vi "programa14.vi"() -> ()   [LabVIEW 2011]
panel:
  in  "stop":bool
  out "Velocidad":i32(knob) scale=0.0..180.0
  in  "Reducir":bool
  in  "Aumentar":bool
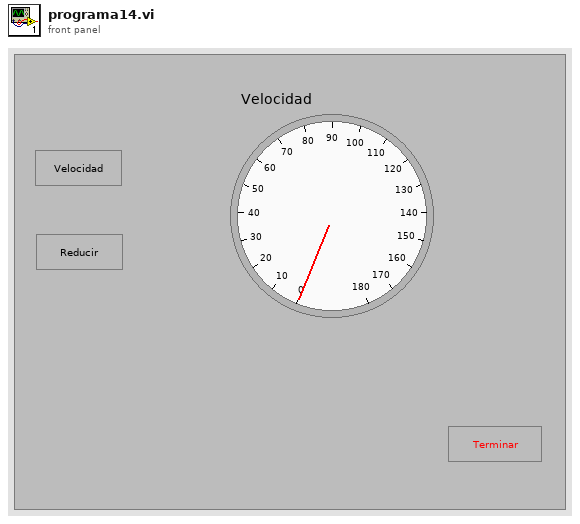
[diagram p1: front panel]
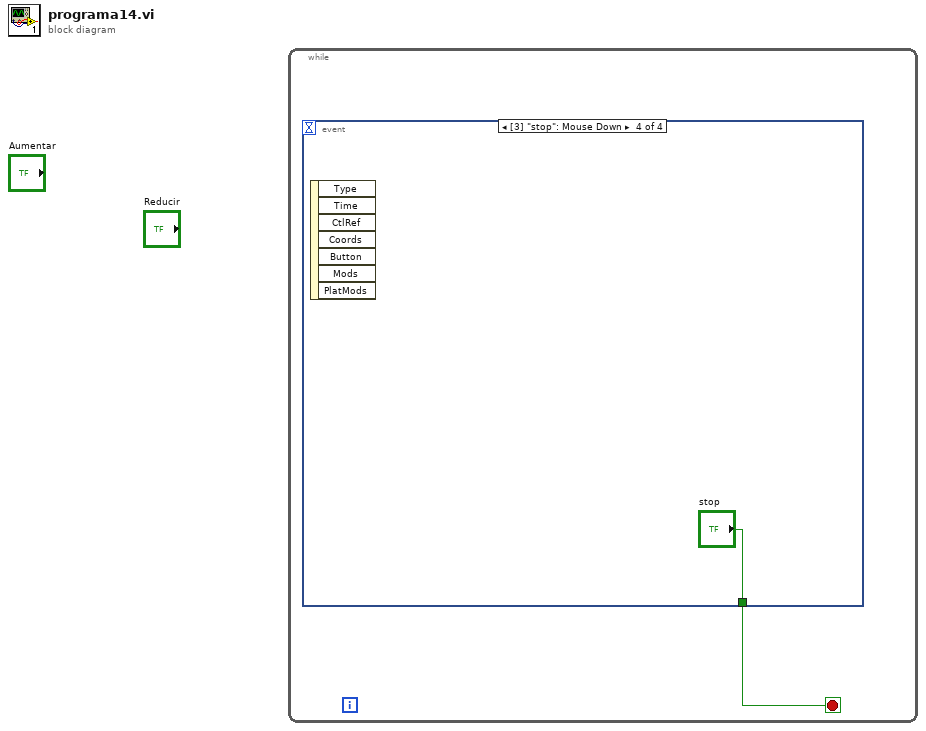
[diagram p0: block diagram]
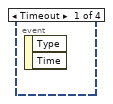
[diagram p2: hidden frame]
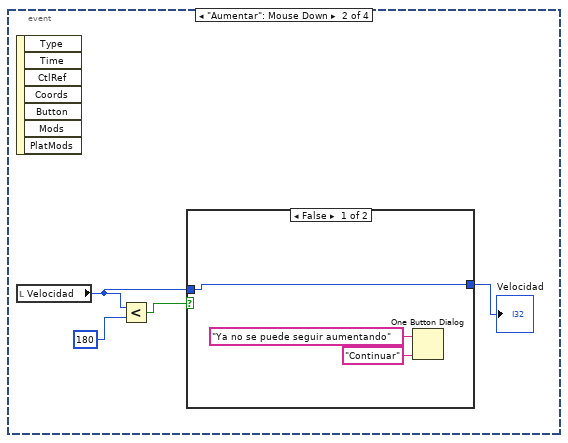
[diagram p3: hidden frame]
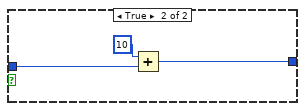
[diagram p4: hidden frame]
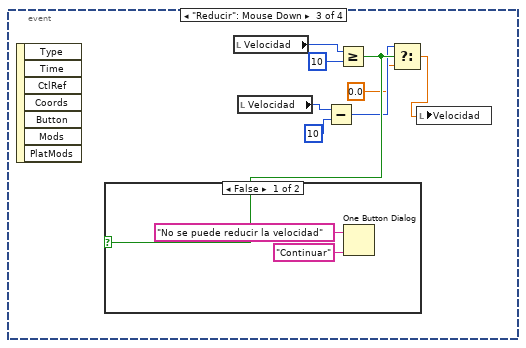
[diagram p5: hidden frame]
diagram:
  n1 = while {
    stop <- w1 stop-if-true
    n2 = event shown="[3] \"stop\": Mouse Down" {
      selector: _ -> [_ _ _ _]
      dyn-events: _ -> [_ _ _ _]
      timeout: _ -> [_ _ _ _]
      tunnel: [_ _ _ "stop"] -> w1
      event Timeout {
        n3 = event-data() -> ()  [unwired: 1 in, 2 out]
      }
      event "Aumentar": Mouse Down {
        n4 = event-data() -> ()  [unwired: 1 in, 7 out]
        n5 = local read "Velocidad"() -> (w4:i32)
        n6 = Less?(x=w4, y=180) -> (x < y?=w3:bool)
        n7 = case shown="False" w3 {
          tunnel: [w8 w10] -> w5
          tunnel: w4 -> [w8 w9]
          frame False {
            n8 = One Button Dialog(message="Ya no se puede seguir aumentando", button name ("OK")="Continuar") -> ()  [unwired: 1 out]
          }
          frame True {
            n9 = Add(x=10, y=w9) -> (x+y=w10:i32)
          }
        }
        "Velocidad" <- w5
      }
      event "Reducir": Mouse Down {
        n10 = event-data() -> ()  [unwired: 1 in, 7 out]
        n11 = local read "Velocidad"() -> (w15:i32)
        n12 = local read "Velocidad"() -> (w18:i32)
        n13 = Subtract(x=w18, y=10) -> (x-y=w13:i32)
        n14 = Greater Or Equal?(x=w15, y=10) -> (x >= y?=w14:bool)
        n15 = case shown="False" w14 {
          frame False {
            n16 = One Button Dialog(message="No se puede reducir la velocidad", button name ("OK")="Continuar") -> ()  [unwired: 1 out]
          }
          frame True {
          }
        }
        n17 = Select(t=w13, s=w14, f=0.0 ("t")) -> (s? t:f=w16:dbl)
        n18 = local write "Velocidad"(w16) -> ()
      }
      event "stop": Mouse Down {
        n19 = event-data() -> ()  [unwired: 1 in, 7 out]
      }
    }
  }
